vi "Self-Cal.vi"(8 "error in":errorcluster caption="error in (no error)", 11 "Resource":string) -> (0 "error out":errorcluster, 3 "Result":string)   [LabVIEW 2020, in "NI SysCfg.lvlib"]
uses:
  NI SysCfg.lvlib
  <vilib>/nisyscfg/Close (Hardware).vi
  <vilib>/nisyscfg/Close (System).vi
  <vilib>/nisyscfg/nisyscfg.lvlib
  <resource>/objmgr/niMIDebugSession.rc
  <resource>/objmgr/nicontrollersysapi.rc
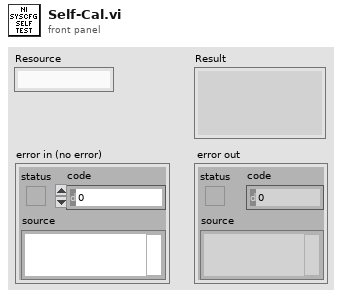
[diagram p1: front panel]
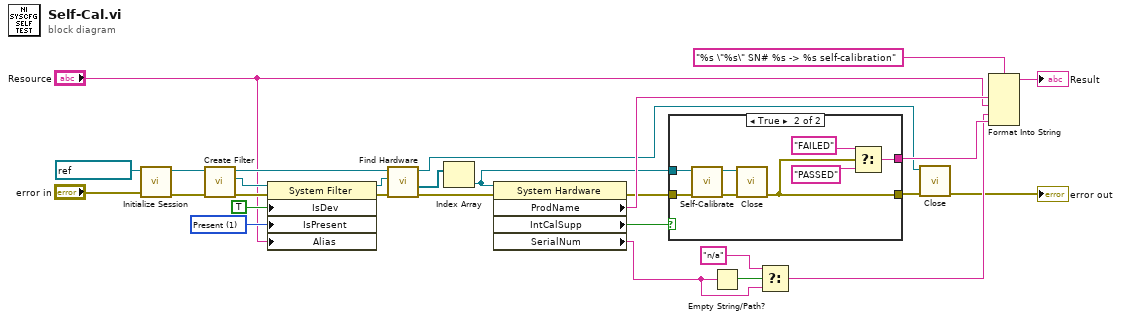
[diagram p0: block diagram]
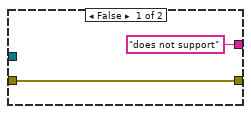
[diagram p2: hidden frame]
diagram:
  w25 = 1 items=["Initializing"=-2, "Unknown"=-1, "Not Present"=0, "Present"=1] ("Devices & Chassis:Is Present")
  n1 = call <vilib>:"Initialize Session.vi"("error in (no error)"="error in", "Target (localhost)"=refnum<k21> "localhost") -> ("error out"=w24:errorcluster, "Session out"=w23:refnum<k21>)  [unwired: 8 in]
  n2 = call <vilib>:"Create Filter.vi"("error in (no error)"=w24, "Session in"=w23) -> ("error out"=w15:errorcluster, "Filter out"=w16:refnum<k20>, "Session out"=w19:refnum<k21>)  [unwired: 7 in]
  n3 = property class="System Filter"(reference=w16, error in=w15, "IsDev"=TRUE ("Is Device"), "IsPresent"=w25, "Alias"="Resource") -> (reference out=w18:refnum<k20>, error out=w17:errorcluster)
  n4 = call <vilib>:"Find Hardware.vi"("error in (no error)"=w17, "Filter in"=w18, "Session in"=w19) -> ("error out"=w11:errorcluster, "Resources out"=w21:refnum<k20>[], "Session out"=w1:refnum<k21>)  [unwired: 5 in, 1 out]
  n5 = Index Array(array=w21) -> (element=w22:refnum<k20>)  [unwired: 1 in]
  n6 = property class="System Hardware"(reference=w22, error in=w11) -> (error out=w12:errorcluster, "ProdName"=w27:string, "IntCalSupp"=w4:bool, "SerialNum"=w5:string)  [unwired: 1 out]
  n7 = case shown="True" w4 {
    tunnel: [w30 w31] -> w3
    tunnel: w22 -> [_ w36]
    tunnel: w12 -> [w30 w33]
    tunnel: ["does not support" ("format string") w32] -> w9
    frame False {
    }
    frame True {
      n8 = call <vilib>:"Self-Calibrate.vi"("error in (no error)"=w33, "Resource in"=w36) -> ("error out"=w34:errorcluster, "Resource out"=w35:refnum<k20>)  [unwired: 7 in, 1 out]
      n9 = call-poly <vilib>:"Close.vi"("error in (no error)"=w34, "Resource in"=w35) -> ("error out"=w31:errorcluster)  [unwired: 9 in]
      n10 = Select(t="FAILED" ("format string"), s=w31, f="PASSED" ("format string")) -> (s? t:f=w32:string)
    }
  }
  n11 = Empty String/Path?(string/path=w5) -> (empty?=w8:bool)
  n12 = Select(t="n/a", s=w8, f=w5) -> (s? t:f=w6:string)
  n13 = call-poly <vilib>:"Close.vi"("error in (no error)"=w3, "Session in"=w1) -> ("error out"=→"error out":errorcluster)  [unwired: 9 in]
  n14 = Format Into String(format string="%s \"%s\" SN# %s -> %s self-calibration", w27, "Resource", w6, w9) -> (resulting string=→"Result":string)  [unwired: 2 in, 1 out]
